vi "loadDataNodeBegin.vi"(8 "error in (no error)":errorcluster, 10 "XML Refnum in":refnum<file>, 11 "PWM in":refnum<class "PWM.lvclass">) -> (0 "error out":errorcluster, 2 "XML Refnum out":refnum<file>, 3 "PWM out":refnum<class "PWM.lvclass">)   [LabVIEW 2014, in "PWM.lvclass"]
doc: "Part of the file loading process. Occurs at the beginning of a node being loaded. Loads the common xceDataNode data name and description."
uses:
  PWM.lvclass
  Parameters/Parameters.lvclass
  Channel/Channel.lvclass
  XML Parser/XML Parser.lvclass
  xCE/xceNode/xceNode.lvclass
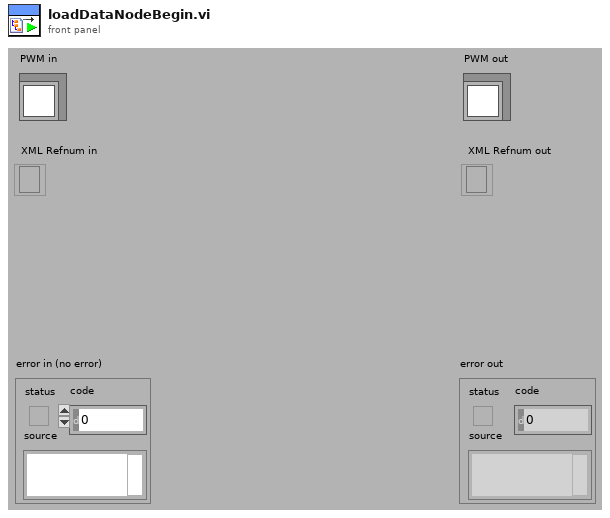
[diagram p1: front panel]
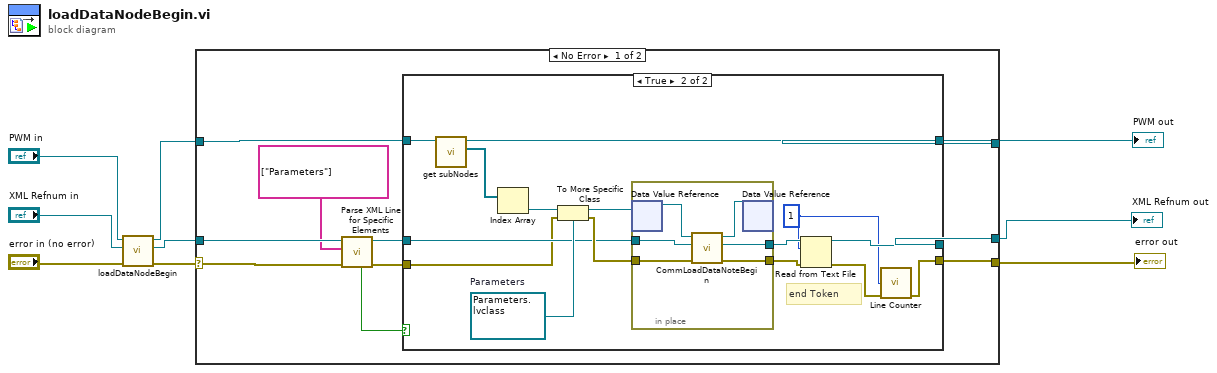
[diagram p0: block diagram]
diagram:
  n1 = call-parent "loadDataNodeBegin.vi"("error in (no error)"="error in (no error)", "XML Refnum in"="XML Refnum in", "Channel in"="PWM in") -> ("error out"=w6:errorcluster, "XML Refnum out"=w5:refnum<file>, "Channel out"=w4:refnum<class "PWM.lvclass">)  [unwired: 6 in]
  n2 = case shown="No Error" w6 {
    selector: w6 -> [w17 w44]
    tunnel: w5 -> [w19 w45]
    tunnel: w4 -> [w18 w46]
    tunnel: [w16 w46] -> w3
    tunnel: [w15 w45] -> w2
    tunnel: [w14 w44] -> w1
    frame No Error {
      n3 = call "Parse XML Line for Specific Elements.vi"("error in (no error)"=w17, "Elements"=string[] ["Parameters"] ("Token List"), "XML Refnum in"=w19) -> ("error out"=w10:errorcluster, "XML Refnum out"=w11:refnum<file>, "Element Found"=w12:bool)  [unwired: 4 in, 2 out]
      n4 = case shown="True" w12 {
        tunnel: w11 -> [w22 w27]
        tunnel: w10 -> [w20 w26]
        tunnel: w18 -> [w21 w37]
        tunnel: [w21 w32] -> w16
        tunnel: [w22 w31] -> w15
        tunnel: [w20 w23] -> w14
        frame False {
        }
        frame True {
          w30 = refnum<data-value> refnum  # Parameters
          w24 = 1 ("count")
          # "end Token"
          n5 = call "get subNodes.vi"("xceNode in"=w37) -> ("subNodes[]*"=w36:refnum<data-value>[], "xceNode out"=w32:refnum<class "PWM.lvclass">)  [unwired: 8 in, 1 out]
          n6 = Index Array(array=w36) -> (element=w35:refnum<data-value>)  [unwired: 1 in]
          n7 = To More Specific Class(target class=w30, reference=w35, error in=w26) -> (specific class reference=w34:refnum<data-value>, error out=w33:errorcluster)
          n8 = in-place {
            in-place-border: w33 -> [w41]
            in-place-border: w27 -> [w42]
            in-place-border: [w39] -> w29
            in-place-border: [w38] -> w28
            n9 = in-place-dvr #1(w34) -> (w43:refnum<class "Parameters.lvclass">)  [unwired: 1 out]
            n10 = call "CommLoadDataNoteBegin.vi"("error in (no error)"=w41, "XML Refnum in"=w42, "Parameters In"=w43) -> ("error out"=w38:errorcluster, "XML Refnum out"=w39:refnum<file>, "Parameters Out"=w40:refnum<class "Parameters.lvclass">)  [unwired: 6 in]
            n11 = in-place-dvr #1(w40) -> ()  [unwired: 2 out]
          }
          n12 = Read from Text File(file (use dialog)=w29, count=w24, error in=w28) -> (refnum out=w31:refnum<file>, error out=w25:errorcluster)  [unwired: 1 in, 2 out]
          n13 = call "Line Counter.vi"("error in (no error)"=w25, "# of lines to increment (1)"=w24) -> ("error out"=w23:errorcluster)  [unwired: 8 in, 1 out]
        }
      }
    }
    frame Error {
    }
  }
  "error out" <- w1
  "PWM out" <- w3
  "XML Refnum out" <- w2
